vi "Destroy.vi"(8 "Error In":errorcluster, 11 "reference in":refnum<class "Scope Base.lvclass">) -> (0 "Error Out":errorcluster, 3 "reference out":refnum<class "Scope Base.lvclass">)   [LabVIEW 2023, in "Scope Base.lvlib" / "Scope Base.lvclass"]
uses:
  Scope Base.lvclass
  Instrument Base/Instr Base.lvclass
  Scope Base.lvclass/Scope Base.ctl
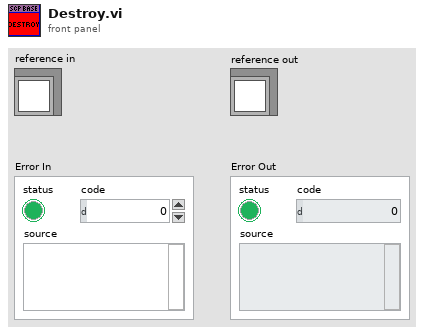
[diagram p1: front panel]
types:
  T1 = typedef "Scope Base.lvlib/Scope Base.lvclass/ObjectAttributes.ctl" = cluster{"Last Waveforms":map{u8, waveform(dbl)}}
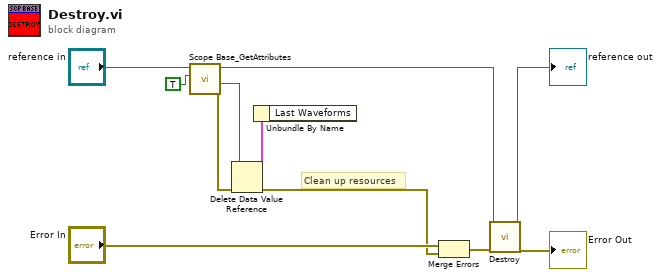
[diagram p0: block diagram]
diagram:
  # "Clean up resources"
  n1 = call "Scope Base_GetAttributes.vi"("OnlyGetDvrReference(False)"=TRUE, "reference in"="reference in") -> ("Error Out"=w9:errorcluster, "DataRef"=w7:refnum<data-value>, "reference out"=w8:refnum<class "Scope Base.lvclass">)  [unwired: 6 in, 1 out]
  n2 = Delete Data Value Reference(data value reference=w7, error in=w9) -> (data value=w1:T1, error out=w5:errorcluster)
  n3 = Unbundle By Name(w1) -> ()  [unwired: 1 out]
  n4 = Merge Errors("Error In", w5) -> (w11:errorcluster)
  n5 = call-parent "Destroy.vi"("Error In"=w11, "reference in"=w8) -> ("Error Out"=→"Error Out":errorcluster, "reference out"=→"reference out":refnum<class "Scope Base.lvclass">)  [unwired: 8 in]
